vi "Compare OTP Against File.vi"(7 "result":u32, 8 "error in (no error)":errorcluster, 9 "resultsFilename":string, 10 "filename":string, 11 "_hResourceContext":u32) -> (0 "error out":errorcluster, 1 "resultsFilename out":string, 2 "filename out":string, 3 "_hResourceContext out":u32, 5 "result out":u32)   [LabVIEW 2013, in "QCAWLAN_DLL.lvlib"]
doc: "QCA_DLL_Export void CompareOTPAgainstFile(HANDLE _hResourceContext, char *filename, char *resultsFilename, unsigned int *result);"
uses:
  QCAWLAN_DLL.lvlib
  QCAWLAN_DLL.dll
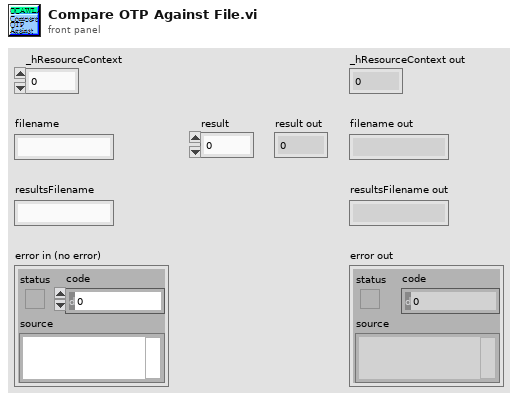
[diagram p1: front panel]
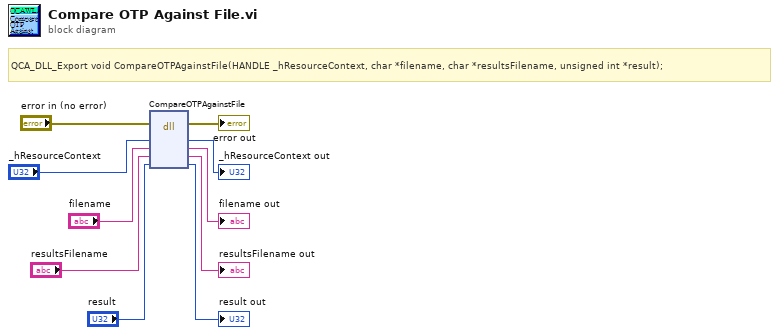
[diagram p0: block diagram]
diagram:
  # "QCA_DLL_Export void CompareOTPAgainstFile(HANDLE _hResourceContext, char *filename, char *resultsFilename, unsigned int *result);"
  n1 = dll-call lib="C:/Users/dave_yao/Desktop/Hitron/QCA9984 WLAN_LV2013/user.lib/QCAWLAN_DLL/QCAWLAN_DLL.*" fn="CompareOTPAgainstFile"(error in="error in (no error)", "_hResourceContext"="_hResourceContext", "filename"="filename", "resultsFilename"="resultsFilename", "result"="result") -> (error out=→"error out":errorcluster, "_hResourceContext"=→"_hResourceContext out":u32, "filename"=→"filename out":string, "resultsFilename"=→"resultsFilename out":string, "result"=→"result out":u32)  [unwired: 3 in, 1 out]
